vi "UpdateBusFromFrontPanel.vi"(8 "ErrorArray In":errorcluster[](array[cluster])) -> (0 "ErrorArray Out":errorcluster[](array[cluster]), 2 "output cluster":T1={"BusNumber"=0, "EvtPluginINIFilePath"=path "", "EvtParams"=[], "EvtConfig"={"UTC Time 0"=timestamp(0 s since 1904-01-01), "Nominal Frequency"=60, "Reporting Rate"=60, "Fsamp"=960, "PosSeq"=FALSE}, "Start Time"=0.0, "End Time"=0.0, "PmuImpairPluginINIFilePath"=path "", "PmuImpairParams "=[["960"], ["8.19"], ["164"]], "PmuImpairConfig"={"FilterType"="", "bPosSeq"=TRUE}, "NetImpPluginINIFilePath"=path "", "NetImpParams"=[], "FlagImpPluginINIFilePath"=path "", "FlagImpParams"=[], "EvtReportArray"=[], "EventSignalArray"=[], "ImpairReportArray"=[], "NetworkTime"=[], "PktLoss"=[], "FlagImpArray"=[], "OutputToFilePluginINIFilePath"=path "", "Output File Path"=path "", "clConfigOptions"={"TIME_BASE"=1000000, "STN"="Bus_1", "IDCODE"=0, "rdoPolRect"=enum."Rectangular", "rdoFloatInt"=enum."Float", "PHUNIT"=1000000, "rdoFreqDfreq"=enum."Float", "CHNAM"=["VA", "VB", "VC", "V+", "IA", "IB", "IC", "I+"], "chkCfg2Prefix"=TRUE}, "AppPluginINIFilePath"=path "", "AppConfig"=variant, "AppOutput"=variant} {"clConfigOptions"."PHUNIT" max=16777216 step=1 format="%08d"; "clConfigOptions"."IDCODE" format="%02x"; "clConfigOptions"."TIME_BASE" max=16777216 step=1 format="%08d"; "ImpairReportArray"."Synx" format="%#_4g"; "EvtReportArray"."Synx" format="%#_4g"; "EvtConfig"."Reporting Rate" items=["10 FPS"=10, "12 FPS"=12, "15 FPS"=15, "20 FPS"=20, "25 FPS"=25, "30 FPS"=30, "50 FPS"=50, "60 FPS"=60]; "EvtConfig"."Nominal Frequency" items=["50 Hz"=50, "60 Hz"=60]}, 3 "Framework.lvlib:Bus.lvclass":refnum<class "Bus.lvclass">)   [LabVIEW 2014, in "Framework.lvlib"]
doc: "Update each module within a bus from the data on the front panel."
uses:
  Framework.lvlib
  Bus_class/Public/TypeDefs/clBusData.ctl
  TypeDefs/clEventConfig.ctl
  Modules/PmuImpairPlugins/PmuImpairPluginBase_class/TypeDefs/clImpairConfig.ctl
  Modules/EventPlugins/EventPluginBaseClass/TypeDefs/clEvtReportArray.ctl
  Modules/EventPlugins/EventPluginBaseClass/TypeDefs/clEvtReport.ctl
  Modules/EventPlugins/EventPluginBaseClass/TypeDefs/dblEvtSignalArray.ctl
  Modules/NetworkImpairmentModule/PublicAPI/Arguments/Broadcasts/dblNetworkTime.ctl
  Modules/NetworkImpairmentModule/PublicAPI/Arguments/Broadcasts/dblPktLoss.ctl
  Modules/FlagImpairModule/PublicAPI/Arguments/Broadcasts/ui32FlagImpairmentArray.ctl
  Modules/OutputToFilePlugins/OutputToFileBasePlugin/Typedefs/PmuCfgOpt.ctl
  Bus_class/Bus.lvclass
  Config_class/Config.lvclass/Config.ctl
  Config_class/Accessors/Read PARTF Root Directory.vi
  Modules/EventPlugins/EventPluginBaseClass/EventPluginBaseClass.lvclass
  Modules/NetworkImpairmentModule/NetworkImpairmentModule.lvlib
  Modules/FlagImpairModule/FlagImpairModule.lvlib
  Modules/OutputToFilePlugins/OutputToFileBasePlugin/OutputToFileBasePlugin.lvclass
  Modules/PmuImpairPlugins/PmuImpairPluginBase_class/PmuImpairPluginBase.lvclass
  Config_class/Config.lvclass
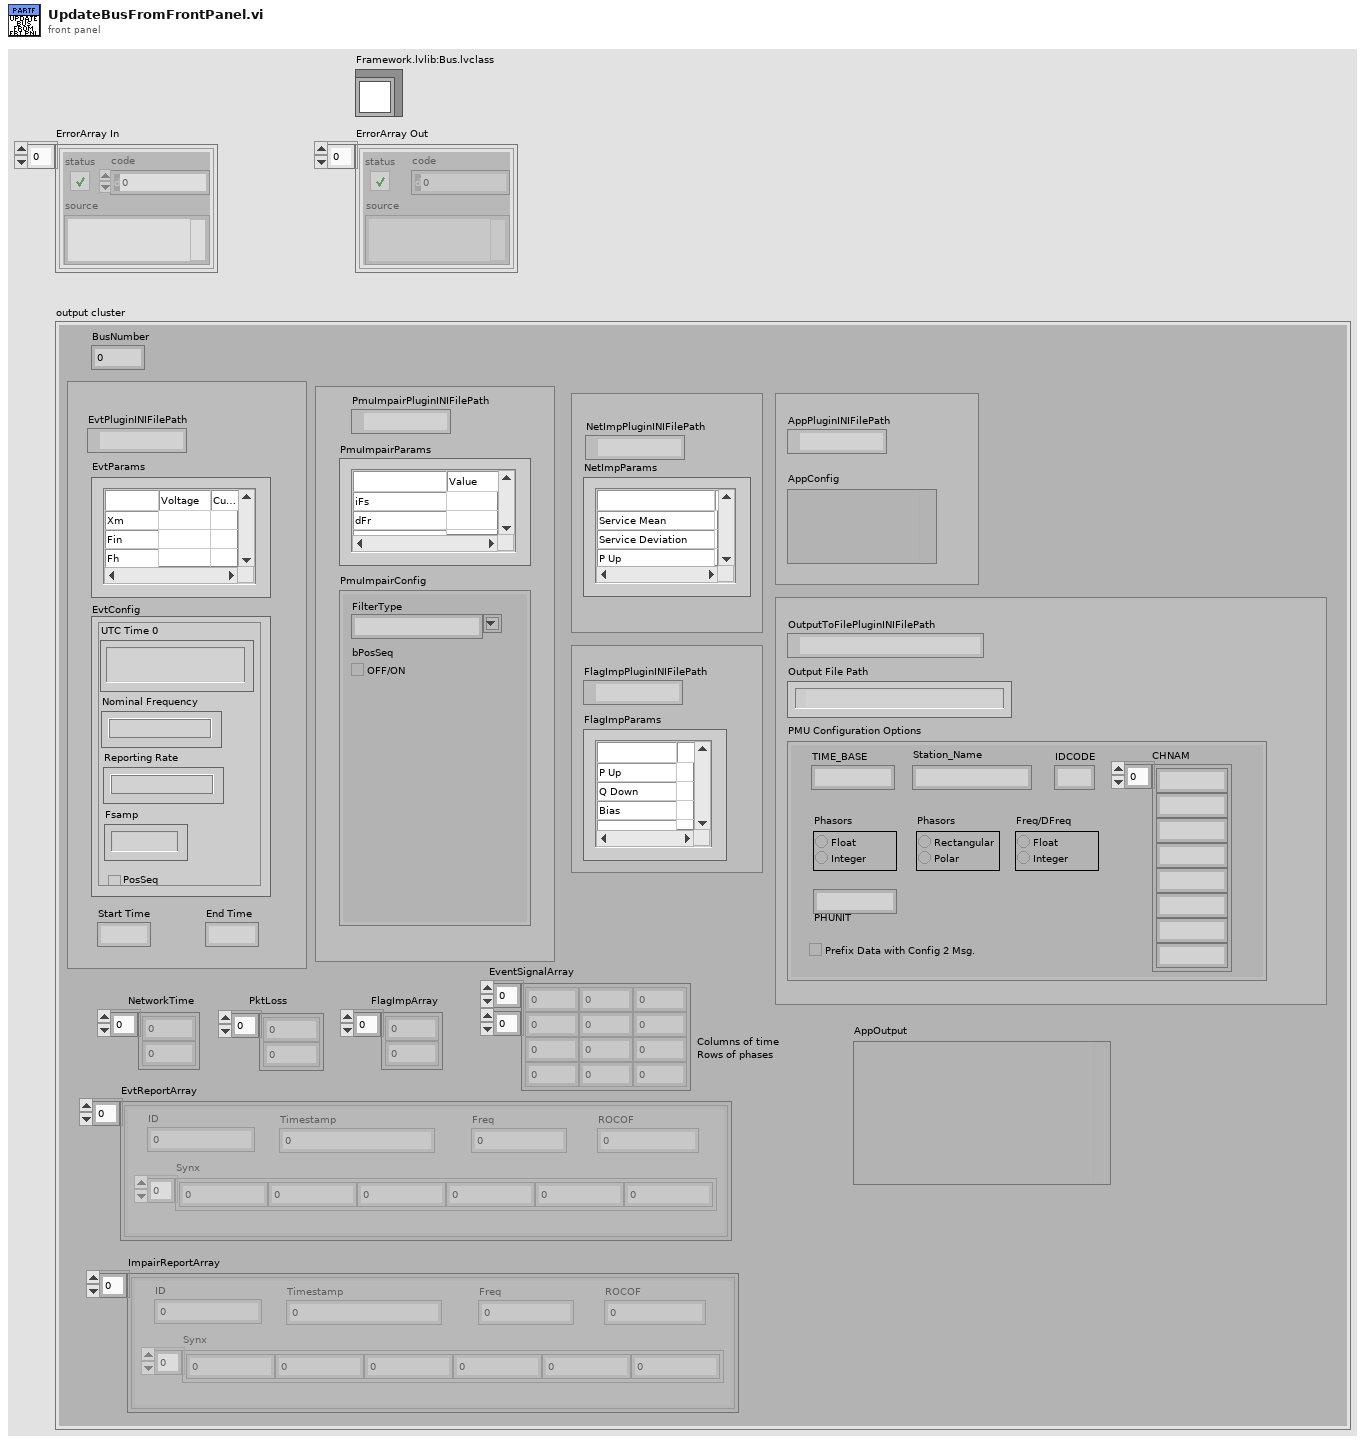
[diagram p1: front panel]
types:
  T1 = typedef "Bus_class.lvlib/Bus.lvclass/clBusData.ctl" = cluster{"BusNumber":u8, "EvtPluginINIFilePath":path, "EvtParams":string[][], "EvtConfig":T2, "Start Time":dbl, "End Time":dbl, "PmuImpairPluginINIFilePath":path, "PmuImpairParams ":string[][], "PmuImpairConfig":T3, "NetImpPluginINIFilePath":path, "NetImpParams":string[][], "FlagImpPluginINIFilePath":path, "FlagImpParams":string[][], "EvtReportArray":T4, "EventSignalArray":T6, "ImpairReportArray":T4, "NetworkTime":T7, "PktLoss":T8, "FlagImpArray":T9, "OutputToFilePluginINIFilePath":path, "Output File Path":path, "clConfigOptions":T10, "AppPluginINIFilePath":path, "AppConfig":variant, "AppOutput":variant}
  T2 = typedef "Framework.lvlib/clEventConfig.ctl" = cluster{"UTC Time 0":timestamp, "Nominal Frequency":u16, "Reporting Rate":u16, "Fsamp":u32, "PosSeq":bool}
  T3 = typedef "PmuImpairPlugins.lvlib/PmuImpairPluginBase.lvclass/clImpairConfig.ctl" = cluster{"FilterType":string, "bPosSeq":bool}
  T4 = typedef "EventPlugins.lvlib/EventPluginBaseClass.lvclass/clEvtReportArray.ctl" = T5[]
  T5 = typedef "EventPlugins.lvlib/EventPluginBaseClass.lvclass/clEvtReport.ctl" = cluster{"Timestamp":dbl, "Synx":cdb[], "Freq":dbl, "ROCOF":dbl, "ID":i16}
  T6 = typedef "EventPlugins.lvlib/EventPluginBaseClass.lvclass/dblEvtSignalArray.ctl" = dbl[][]
  T7 = typedef "NetworkImpairmentModule.lvlib/dblNetworkTime.ctl" = dbl[]
  T8 = typedef "NetworkImpairmentModule.lvlib/dblPktLoss.ctl" = dbl[]
  T9 = typedef "FlagImpairModule.lvlib/ui32FlagImpairmentArray.ctl" = u32[]
  T10 = typedef "OutputToFilePlugins.lvlib/OutputToFileBasePlugin.lvclass/PmuCfgOpt.ctl" = cluster{"TIME_BASE":u64, "STN":string, "IDCODE":u16, "rdoPolRect":enum32{"Rectangular", "Polar"}, "rdoFloatInt":enum32{"Float", "Integer"}, "PHUNIT":u64, "rdoFreqDfreq":enum32{"Float", "Integer"}, "CHNAM":string[], "chkCfg2Prefix":bool}
  T11 = typedef "Framework.lvlib/clFrontPanelControlRefs.ctl" = cluster{"TestFilePathRef":refnum<vi>, "BusNumberRef":refnum<vi>, "NumberOfBusesRef":refnum<vi>, "EvtTypeRef":refnum<vi>, "EvtParamsRef":refnum<vi>, "EvtConfigRef":refnum<vi>, "StartTimeRef":refnum<vi>, "EndTimeRef":refnum<vi>, "PmuImpairTypeRef":refnum<vi>, "PmuImpairParamsRef":refnum<vi>, "NetImpairParamsRef":refnum<vi>, "FlagImpairTypeRef":refnum<vi>, "FlagImpairParamsRef":refnum<vi>, "NetImpairTypeRef":refnum<vi>, "OutputFileType":refnum<vi>, "PmuImpairConfigRef":refnum<vi>, "AppTypeRef":refnum<vi>, "ScriptPathRef":refnum<vi>, "ShowPanels?":refnum<vi>}
  T12 = typedef "Framework.lvlib/Config.lvclass/RootDir.ctl" = cluster{"pathRootDir":path, "btnOutPath":bool, "OutDir":string, "btnOpenOutputDir":bool, "ScriptDir":string, "btnOpenScriptDir":bool, "TestDir":string, "btnOpenTestDir":bool}
  T13 = typedef "Framework.lvlib/clFrameworkData.ctl" = cluster{"EvtINIFilePaths":path[], "BusClassInstances":refnum<class "Bus.lvclass">[], "PmuImpairINIFilePaths":path[], "FlagImpairINIFilePaths":path[], "NetImpairINIFilePaths":path[], "OutputToFileINIFilePaths":path[], "AppINIFilePaths":path[], "AppModuleID":i32, "OutputToFileID":i32}
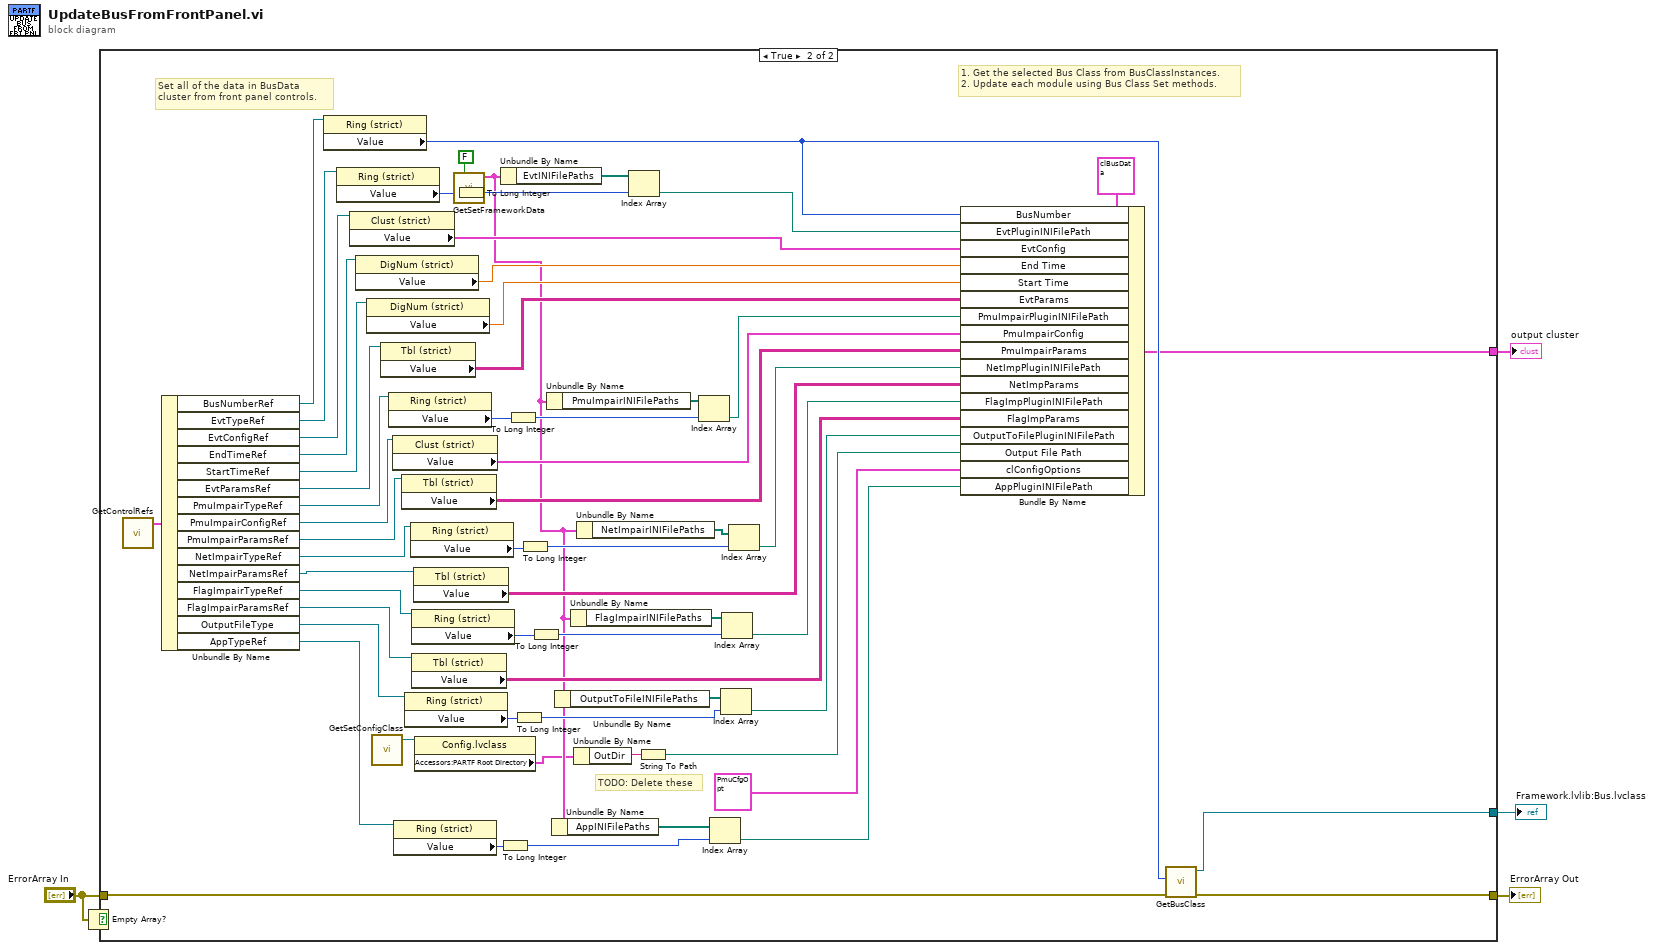
[diagram p0: block diagram]
diagram:
  n1 = Empty Array?(array="ErrorArray In") -> (empty?=w3:bool)
  n2 = case shown="True" w3 {
    tunnel: "ErrorArray In" -> [w6 w67]
    tunnel: [w6 w14] -> w5
    tunnel: [_ w16] -> w2
    tunnel: [_ w15] -> w1
    frame False {
    }
    frame True {
      # "TODO: Delete these"
      # "1. Get the selected Bus Class from BusClassInstances.\n2. Update each module using Bus Class Set methods."
      # "Set all of the data in BusData \ncluster from front panel controls."
      n3 = call "GetControlRefs.vi"() -> ("clControlRefs Out"=w7:T11)  [unwired: 11 in]
      n4 = Unbundle By Name(w7) -> ("BusNumberRef"=w66:refnum<vi>, "EvtTypeRef"=w60:refnum<vi>, "EvtConfigRef"=w58:refnum<vi>, "EndTimeRef"=w56:refnum<vi>, "StartTimeRef"=w55:refnum<vi>, "EvtParamsRef"=w54:refnum<vi>, "PmuImpairTypeRef"=w48:refnum<vi>, "PmuImpairConfigRef"=w46:refnum<vi>, "PmuImpairParamsRef"=w44:refnum<vi>, "NetImpairTypeRef"=w31:refnum<vi>, "NetImpairParamsRef"=w32:refnum<vi>, "FlagImpairTypeRef"=w33:refnum<vi>, "FlagImpairParamsRef"=w34:refnum<vi>, "OutputFileType"=w25:refnum<vi>, "AppTypeRef"=w12:refnum<vi>)
      n5 = property class="Ring (strict)"(reference=w66) -> ("Value"=w52:u8)  [unwired: 1 in, 2 out]
      n6 = property class="Ring (strict)"(reference=w60) -> ("Value"=w61:u16)  [unwired: 1 in, 2 out]
      n7 = property class="Clust (strict)"(reference=w58) -> ("Value"=w57:T2)  [unwired: 1 in, 2 out]
      n8 = property class="DigNum (strict)"(reference=w56) -> ("Value"=w42:dbl)  [unwired: 1 in, 2 out]
      n9 = property class="DigNum (strict)"(reference=w55) -> ("Value"=w41:dbl)  [unwired: 1 in, 2 out]
      n10 = call "GetSetConfigClass.vi"() -> ("Ref out"=w11:refnum<class "Config.lvclass">)  [unwired: 11 in]
      n11 = property class="Tbl (strict)"(reference=w54) -> ("Value"=w53:string[][])  [unwired: 1 in, 2 out]
      n12 = property class="Ring (strict)"(reference=w48) -> ("Value"=w51:u16)  [unwired: 1 in, 2 out]
      n13 = property class="Clust (strict)"(reference=w46) -> ("Value"=w45:T3)  [unwired: 1 in, 2 out]
      n14 = property class="Ring (strict)"(reference=w12) -> ("Value"=w21:u16)  [unwired: 1 in, 2 out]
      n15 = property class="Tbl (strict)"(reference=w44) -> ("Value"=w43:string[][])  [unwired: 1 in, 2 out]
      n16 = property class="Ring (strict)"(reference=w25) -> ("Value"=w24:u16)  [unwired: 1 in, 2 out]
      n17 = property class="Ring (strict)"(reference=w31) -> ("Value"=w29:u16)  [unwired: 1 in, 2 out]
      n18 = property class="Ring (strict)"(reference=w33) -> ("Value"=w37:u16)  [unwired: 1 in, 2 out]
      n19 = property class="Tbl (strict)"(reference=w34) -> ("Value"=w35:string[][])  [unwired: 1 in, 2 out]
      n20 = property class="Tbl (strict)"(reference=w32) -> ("Value"=w40:string[][])  [unwired: 1 in, 2 out]
      n21 = property class="Config.lvclass"(reference=w11) -> ("Accessors:PARTF Root Directory"=w10:T12)  [unwired: 1 in, 2 out]
      n22 = call "GetSetFrameworkData.vi"("Set (F)"=FALSE) -> ("clFrameworkData Out"=w20:T13)  [unwired: 10 in]
      n23 = To Long Integer(number=w61) -> (32bit integer=w64:i32)
      n24 = To Long Integer(number=w21) -> (32bit integer=w18:i32)
      n25 = Unbundle By Name(w20) -> ("EvtINIFilePaths"=w63:path[])
      n26 = To Long Integer(number=w51) -> (32bit integer=w49:i32)
      n27 = To Long Integer(number=w24) -> (32bit integer=w23:i32)
      n28 = To Long Integer(number=w29) -> (32bit integer=w28:i32)
      n29 = To Long Integer(number=w37) -> (32bit integer=w39:i32)
      n30 = Unbundle By Name(w20) -> ("PmuImpairINIFilePaths"=w50:path[])
      n31 = Unbundle By Name(w20) -> ("AppINIFilePaths"=w19:path[])
      n32 = Unbundle By Name(w20) -> ("OutputToFileINIFilePaths"=w26:path[])
      n33 = Unbundle By Name(w20) -> ("FlagImpairINIFilePaths"=w38:path[])
      n34 = Unbundle By Name(w10) -> ("OutDir"=w9:string)
      n35 = Unbundle By Name(w20) -> ("NetImpairINIFilePaths"=w30:path[])
      n36 = Index Array(array=w63, index=w64) -> (element=w59:path)
      n37 = String To Path(string=w9) -> (path=w8:path)
      n38 = Index Array(array=w50, index=w49) -> (element=w47:path)
      n39 = Index Array(array=w19, index=w18) -> (element=w17:path)
      n40 = Index Array(array=w26, index=w23) -> (element=w22:path)
      n41 = Index Array(array=w38, index=w39) -> (element=w36:path)
      n42 = Index Array(array=w30, index=w28) -> (element=w27:path)
      n43 = Bundle By Name(cluster=T1 {"BusNumber"=0, "EvtPluginINIFilePath"=path "", "EvtParams"=[], "EvtConfig"={"UTC Time 0"=timestamp(0 s since 1904-01-01), "Nominal Frequency"=60, "Reporting Rate"=60, "Fsamp"=960, "PosSeq"=FALSE}, "Start Time"=0.0, "End Time"=0.0, "PmuImpairPluginINIFilePath"=path "", "PmuImpairParams "=[["960"], ["8.19"], ["164"]], "PmuImpairConfig"={"FilterType"="", "bPosSeq"=TRUE}, "NetImpPluginINIFilePath"=path "", "NetImpParams"=[], "FlagImpPluginINIFilePath"=path "", "FlagImpParams"=[], "EvtReportArray"=[], "EventSignalArray"=[], "ImpairReportArray"=[], "NetworkTime"=[], "PktLoss"=[], "FlagImpArray"=[], "OutputToFilePluginINIFilePath"=path "", "Output File Path"=path "", "clConfigOptions"={"TIME_BASE"=1000000, "STN"="Bus_1", "IDCODE"=0, "rdoPolRect"=enum."Rectangular", "rdoFloatInt"=enum."Float", "PHUNIT"=1000000, "rdoFreqDfreq"=enum."Float", "CHNAM"=["VA", "VB", "VC", "V+", "IA", "IB", "IC", "I+"], "chkCfg2Prefix"=TRUE}, "AppPluginINIFilePath"=path "", "AppConfig"=variant, "AppOutput"=variant} ("clBusData"), "BusNumber"=w52, "EvtPluginINIFilePath"=w59, "EvtConfig"=w57, "End Time"=w42, "Start Time"=w41, "EvtParams"=w53, "PmuImpairPluginINIFilePath"=w47, "PmuImpairConfig"=w45, "PmuImpairParams"=w43, "NetImpPluginINIFilePath"=w27, "NetImpParams"=w40, "FlagImpPluginINIFilePath"=w36, "FlagImpParams"=w35, "OutputToFilePluginINIFilePath"=w22, "Output File Path"=w8, "clConfigOptions"=T10 {"TIME_BASE"=1000000, "STN"="Bus_1", "IDCODE"=0, "rdoPolRect"=enum."Rectangular", "rdoFloatInt"=enum."Float", "PHUNIT"=1000000, "rdoFreqDfreq"=enum."Float", "CHNAM"=["VA", "VB", "VC", "V+", "IA", "IB", "IC", "I+"], "chkCfg2Prefix"=TRUE}, "AppPluginINIFilePath"=w17) -> (w16:T1)
      n44 = call "GetBusClass.vi"("ErrorArray In"=w67, "BusNumber"=w52) -> ("ErrorArray Out"=w14:errorcluster[], "Framework.lvlib:Bus.lvclass"=w15:refnum<class "Bus.lvclass">)  [unwired: 8 in]
    }
  }
  "ErrorArray Out" <- w5
  "output cluster" <- w2
  "Framework.lvlib:Bus.lvclass" <- w1
